vi "CRYCalcu Arithmetic Curve.vi"(4 "dB ref":dbl format="%#_6p", 6 "B data for units":T1={"Name"="", "Curve"=[], "X data"=1, "Y data"=1, "Z data"=1, "X axis"=0, "Y axis"=1, "Z axis"=1, "X unit"="Hz", "Y unit"="", "Z unit"="deg.", "X dB ref"=1.0, "Y dB ref"=1.0, "Z dB ref"=1.0, "single val"=FALSE, "protected"=FALSE, "display X"=TRUE, "display Y"=TRUE, "display Z"=TRUE, "Test Info"="", "Step No."=0, "Plot Settings"={"Color"=0, "Interpolation"=0, "Point Style"=0, "Line Style"=0, "Point Color"=0, "Line Width"=0, "Bar Plot Style"=0, "Fill To"=0}, "AutoProtect"=FALSE} {"Z data" items=["dB", "Lin"]; "X data" items=["dB", "Lin"]; "Y data" items=["dB", "Lin"]; "Z dB ref" format="%.1f"; "Z axis" items=["Log", "Lin"]; "X dB ref" format="%.1f"; "X axis" items=["Log", "Lin"]; "Y axis" items=["Log", "Lin"]; "Y dB ref" format="%.1f"; "Curve"."z" format="%.2f"; "Curve"."y" format="%.2f"; "Curve"."x" format="%.2f"}, 7 "A data for units":T1={"Name"="", "Curve"=[], "X data"=1, "Y data"=1, "Z data"=1, "X axis"=0, "Y axis"=1, "Z axis"=1, "X unit"="Hz", "Y unit"="", "Z unit"="deg.", "X dB ref"=1.0, "Y dB ref"=1.0, "Z dB ref"=1.0, "single val"=FALSE, "protected"=FALSE, "display X"=TRUE, "display Y"=TRUE, "display Z"=TRUE, "Test Info"="", "Step No."=0, "Plot Settings"={"Color"=0, "Interpolation"=0, "Point Style"=0, "Line Style"=0, "Point Color"=0, "Line Width"=0, "Bar Plot Style"=0, "Fill To"=0}, "AutoProtect"=FALSE} {"Z data" items=["dB", "Lin"]; "X data" items=["dB", "Lin"]; "Y data" items=["dB", "Lin"]; "Z dB ref" format="%.1f"; "Z axis" items=["Log", "Lin"]; "X dB ref" format="%.1f"; "X axis" items=["Log", "Lin"]; "Y axis" items=["Log", "Lin"]; "Y dB ref" format="%.1f"; "Curve"."z" format="%.2f"; "Curve"."y" format="%.2f"; "Curve"."x" format="%.2f"}, 8 "Curve B":cluster{"x":dbl, "y":dbl, "z":dbl}[](array[cluster]) {"z" format="%.2f"; "y" format="%.2f"; "x" format="%.2f"}, 9 "operator":u16(ring) items=["+", "--", "x", "/"], 10 "Work in":u16(slide), 11 "Curve A":cluster{"x":dbl, "y":dbl, "z":dbl}[](array[cluster]) {"z" format="%.2f"; "y" format="%.2f"; "x" format="%.2f"}) -> (2 "Result":cluster{"x":dbl, "y":dbl, "z":dbl}[](array[cluster]) {"z" format="%.2f"; "y" format="%.2f"; "x" format="%.2f"})   [LabVIEW 2013]
uses:
  Typedef Control/CRYData Cluster.ctl
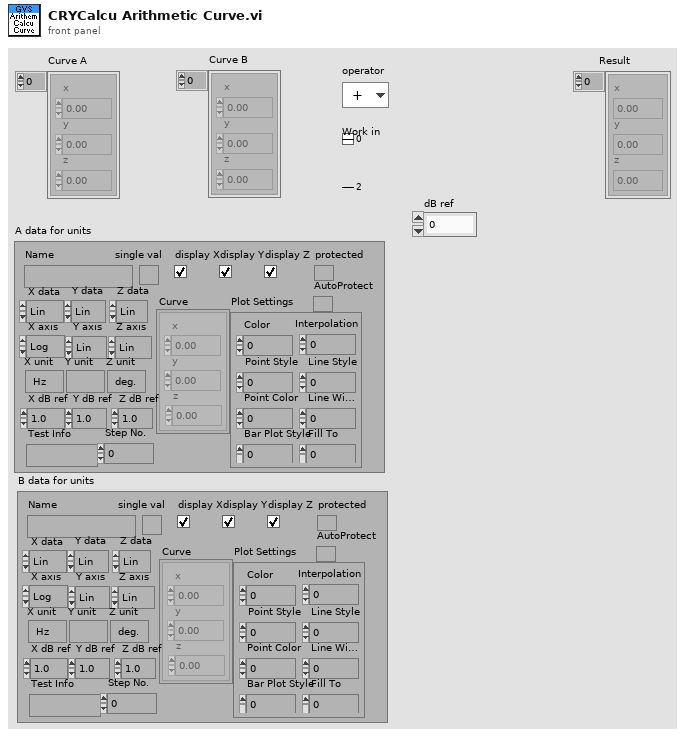
[diagram p1: front panel]
types:
  T1 = typedef "CRYData Cluster.ctl" = cluster{"Name":string, "Curve":cluster{"x":dbl, "y":dbl, "z":dbl}[], "X data":u16, "Y data":u16, "Z data":u16, "X axis":u16, "Y axis":u16, "Z axis":u16, "X unit":string, "Y unit":string, "Z unit":string, "X dB ref":dbl, "Y dB ref":dbl, "Z dB ref":dbl, "single val":bool, "protected":bool, "display X":bool, "display Y":bool, "display Z":bool, "Test Info":string, "Step No.":i32, "Plot Settings":cluster{"Color":u32, "Interpolation":u8, "Point Style":u8, "Line Style":u8, "Point Color":u32, "Line Width":u8, "Bar Plot Style":u8, "Fill To":i16}, "AutoProtect":bool}
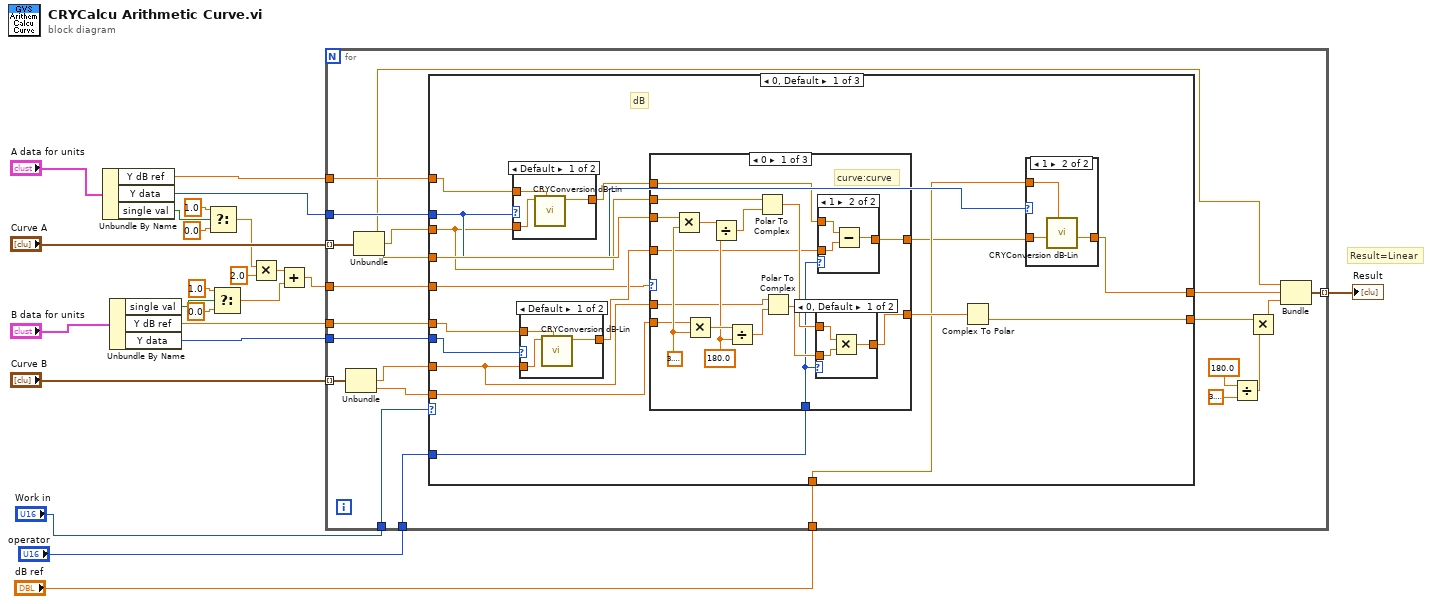
[diagram p0: block diagram]
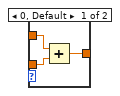
[diagram p2: hidden frame]
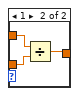
[diagram p3: hidden frame]
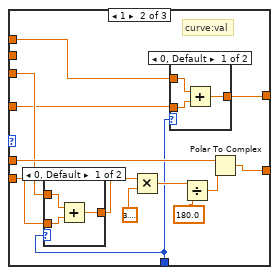
[diagram p4: hidden frame]
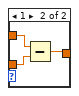
[diagram p5: hidden frame]
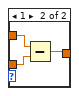
[diagram p6: hidden frame]
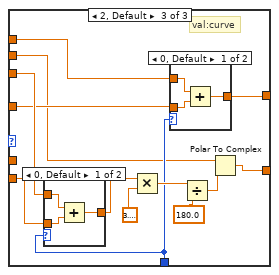
[diagram p7: hidden frame]
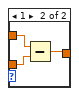
[diagram p8: hidden frame]
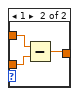
[diagram p9: hidden frame]
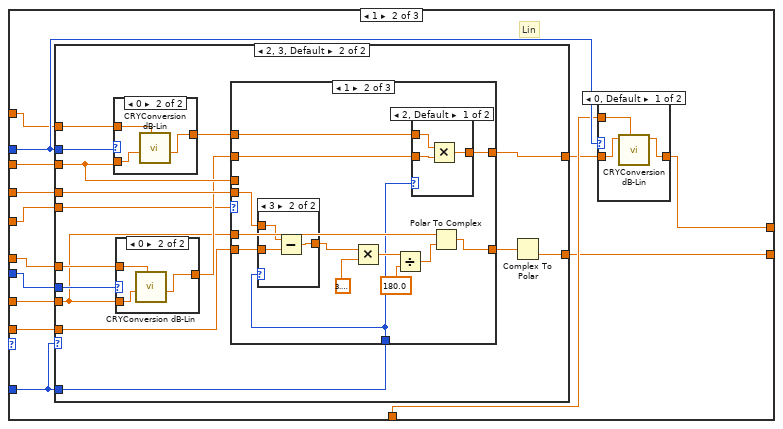
[diagram p13: hidden frame]
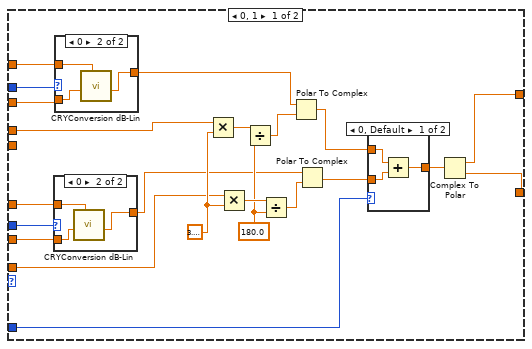
[diagram p14: hidden frame]
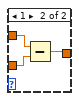
[diagram p15: hidden frame]
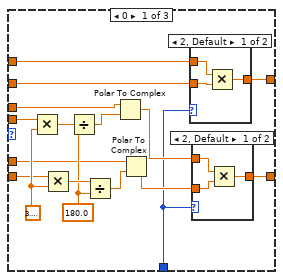
[diagram p18: hidden frame]
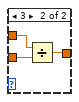
[diagram p19: hidden frame]
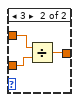
[diagram p20: hidden frame]
diagram:
  # "Result=Linear"
  n1 = Unbundle By Name("A data for units") -> ("Y dB ref"=w17:dbl, "Y data"=w18:u16, "single val"=w13:bool)
  n2 = Unbundle By Name("B data for units") -> ("single val"=w8:bool, "Y dB ref"=w15:dbl, "Y data"=w16:u16)
  n3 = Select(t=1.0, s=w13, f=0.0) -> (s? t:f=w7:dbl)
  n4 = Select(t=1.0, s=w8, f=0.0) -> (s? t:f=w5:dbl)
  n5 = Multiply(x=w7, y=2.0) -> (x*y=w6:dbl)
  n6 = Add(x=w6, y=w5) -> (x+y=w4:dbl)
  n7 = for {
    tunnel: "Curve B" -> [w45] mode=indexing
    tunnel: "Curve A" -> [w44] mode=indexing
    tunnel: [w43] -> w22 mode=indexing
    tunnel: "operator" -> [w42]
    tunnel: "Work in" -> [w41]
    tunnel: w18 -> [w40]
    tunnel: w17 -> [w39]
    tunnel: w16 -> [w38]
    tunnel: w15 -> [w37]
    tunnel: "dB ref" -> [w36]
    tunnel: w4 -> [w25]
    n8 = Unbundle(w45) -> ("y"=w34:dbl, "z"=w28:dbl)  [unwired: 1 out]
    n9 = Unbundle(w44) -> ("x"=w24:dbl, "y"=w35:dbl, "z"=w29:dbl)
    n10 = case shown="0, Default" w41 {
      tunnel: w35 -> [w49 w159 w315]
      tunnel: w34 -> [w51 w160 w314]
      tunnel: w42 -> [w52 w157 w316]
      tunnel: w40 -> [w57 w163 w312]
      tunnel: w39 -> [w56 w162 w318]
      tunnel: w38 -> [w61 w167 w323]
      tunnel: w37 -> [w60 w166 w322]
      tunnel: [w55 w161 w310] -> w33
      tunnel: w36 -> [w50 w158 w313]
      tunnel: w29 -> [w59 w165 w320]
      tunnel: w28 -> [w58 w164 w319]
      tunnel: [w54 w155 w317] -> w26
      tunnel: w25 -> [w47 w154 _]
      frame 0, Default {
        # "dB"
        n11 = case shown="Default" w57 {
          tunnel: w49 -> [w151 w153]
          tunnel: [w150 w153] -> w48
          tunnel: w56 -> [w152 _]
          frame Default {
            n12 = call "CRYConversion dB-Lin.vi"("dB ref."=w152, "Lin In"=w151) -> ("Log Out"=w150:dbl)  [unwired: 4 in, 3 out]
          }
          frame 0 {
          }
        }
        n13 = case shown="Default" w61 {
          tunnel: w51 -> [w147 w149]
          tunnel: [w146 w149] -> w53
          tunnel: w60 -> [w148 _]
          frame Default {
            n14 = call "CRYConversion dB-Lin.vi"("dB ref."=w148, "Lin In"=w147) -> ("Log Out"=w146:dbl)  [unwired: 4 in, 3 out]
          }
          frame 0 {
          }
        }
        n15 = case shown="0" w47 {
          tunnel: [w79 w96 w122] -> w62
          tunnel: w59 -> [w70 w99 w125]
          tunnel: w58 -> [w69 w98 w124]
          tunnel: w53 -> [w68 w94 w120]
          tunnel: [w67 w93 w119] -> w46
          tunnel: w52 -> [w66 w92 w118]
          tunnel: w51 -> [w65 w100 _]
          tunnel: w49 -> [w64 _ w117]
          tunnel: w48 -> [w63 w95 w121]
          frame 0 {
            w71 = 180.0
            w74 = 3.141592653589793
            # "curve:curve"
            n16 = Multiply(x=w70, y=w74) -> (x*y=w72:dbl)
            n17 = Multiply(x=w69, y=w74) -> (x*y=w73:dbl)
            n18 = Divide(x=w72, y=w71) -> (x/y=w75:dbl)
            n19 = Divide(x=w73, y=w71) -> (x/y=w76:dbl)
            n20 = Polar To Complex(1:w75, 2:w64) -> (0:w77:cdb)
            n21 = Polar To Complex(1:w76, 2:w65) -> (0:w78:cdb)
            n22 = case shown="0, Default" w66 {
              tunnel: [w86 w91] -> w79
              tunnel: w78 -> [w87 w89]
              tunnel: w77 -> [w88 w90]
              frame 0, Default {
                n23 = Multiply(x=w88, y=w87) -> (x*y=w86:cdb)
              }
              frame 1 {
                n24 = Divide(x=w90, y=w89) -> (x/y=w91:cdb)
              }
            }
            n25 = case shown="1" w66 {
              tunnel: [w80 w85] -> w67
              tunnel: w68 -> [w81 w83]
              tunnel: w63 -> [w82 w84]
              frame 0, Default {
                n26 = Add(x=w82, y=w81) -> (x+y=w80:dbl)
              }
              frame 1 {
                n27 = Subtract(x=w84, y=w83) -> (x-y=w85:dbl)
              }
            }
          }
          frame 1 {
            # "curve:val"
            n28 = case shown="0, Default" w92 {
              tunnel: [w111 w116] -> w97
              tunnel: w98 -> [w112 w114]
              tunnel: w99 -> [w113 w115]
              frame 0, Default {
                n29 = Add(x=w113, y=w112) -> (x+y=w111:dbl)
              }
              frame 1 {
                n30 = Subtract(x=w115, y=w114) -> (x-y=w116:dbl)
              }
            }
            n31 = Multiply(x=w97, y=3.141592653589793) -> (x*y=w102:dbl)
            n32 = case shown="0, Default" w92 {
              tunnel: [w105 w110] -> w93
              tunnel: w94 -> [w106 w108]
              tunnel: w95 -> [w107 w109]
              frame 0, Default {
                n33 = Add(x=w107, y=w106) -> (x+y=w105:dbl)
              }
              frame 1 {
                n34 = Subtract(x=w109, y=w108) -> (x-y=w110:dbl)
              }
            }
            n35 = Divide(x=w102, y=180.0) -> (x/y=w104:dbl)
            n36 = Polar To Complex(1:w104, 2:w100) -> (0:w96:cdb)
          }
          frame 2, Default {
            # "val:curve"
            n37 = case shown="0, Default" w118 {
              tunnel: [w136 w141] -> w123
              tunnel: w124 -> [w137 w139]
              tunnel: w125 -> [w138 w140]
              frame 0, Default {
                n38 = Add(x=w138, y=w137) -> (x+y=w136:dbl)
              }
              frame 1 {
                n39 = Subtract(x=w140, y=w139) -> (x-y=w141:dbl)
              }
            }
            n40 = Multiply(x=w123, y=3.141592653589793) -> (x*y=w127:dbl)
            n41 = case shown="0, Default" w118 {
              tunnel: [w130 w135] -> w119
              tunnel: w120 -> [w131 w133]
              tunnel: w121 -> [w132 w134]
              frame 0, Default {
                n42 = Add(x=w132, y=w131) -> (x+y=w130:dbl)
              }
              frame 1 {
                n43 = Subtract(x=w134, y=w133) -> (x-y=w135:dbl)
              }
            }
            n44 = Divide(x=w127, y=180.0) -> (x/y=w129:dbl)
            n45 = Polar To Complex(1:w129, 2:w117) -> (0:w122:cdb)
          }
        }
        n46 = Complex To Polar(r * e^(i*theta)=w62) -> (theta=w54:dbl)  [unwired: 1 out]
        n47 = case shown="1" w57 {
          tunnel: w46 -> [w142 w145]
          tunnel: [w142 w144] -> w55
          tunnel: w50 -> [_ w143]
          frame 0, Default {
          }
          frame 1 {
            n48 = call "CRYConversion dB-Lin.vi"("dB ref."=w143, "Log In"=w145) -> ("Lin Out"=w144:dbl)  [unwired: 4 in, 3 out]
          }
        }
      }
      frame 1 {
        # "Lin"
        n49 = case shown="2, 3, Default" w157 {
          tunnel: [w169 w205] -> w155
          tunnel: w167 -> [w181 w218]
          tunnel: w166 -> [w180 w217]
          tunnel: w165 -> [w179 w216]
          tunnel: w164 -> [w178 w215]
          tunnel: w163 -> [w177 w214]
          tunnel: w162 -> [w176 w213]
          tunnel: w160 -> [w175 w209]
          tunnel: w159 -> [w174 w211]
          tunnel: w157 -> [w173 w207]
          tunnel: [w168 w208] -> w156
          tunnel: w154 -> [_ w204]
          frame 0, 1 {
            w182 = 180.0
            w185 = 3.141592653589793
            n50 = case shown="0" w181 {
              tunnel: w175 -> [w196 w198]
              tunnel: [w196 w197] -> w172
              tunnel: w180 -> [_ w199]
              frame Default {
              }
              frame 0 {
                n51 = call "CRYConversion dB-Lin.vi"("dB ref."=w199, "Log In"=w198) -> ("Lin Out"=w197:dbl)  [unwired: 4 in, 3 out]
              }
            }
            n52 = case shown="0" w177 {
              tunnel: w174 -> [w200 w202]
              tunnel: [w200 w201] -> w171
              tunnel: w176 -> [_ w203]
              frame Default {
              }
              frame 0 {
                n53 = call "CRYConversion dB-Lin.vi"("dB ref."=w203, "Log In"=w202) -> ("Lin Out"=w201:dbl)  [unwired: 4 in, 3 out]
              }
            }
            n54 = Multiply(x=w179, y=w185) -> (x*y=w183:dbl)
            n55 = Multiply(x=w178, y=w185) -> (x*y=w184:dbl)
            n56 = Divide(x=w183, y=w182) -> (x/y=w186:dbl)
            n57 = Divide(x=w184, y=w182) -> (x/y=w187:dbl)
            n58 = Polar To Complex(1:w186, 2:w171) -> (0:w188:cdb)
            n59 = Polar To Complex(1:w187, 2:w172) -> (0:w189:cdb)
            n60 = case shown="0, Default" w173 {
              tunnel: [w190 w195] -> w170
              tunnel: w189 -> [w191 w193]
              tunnel: w188 -> [w192 w194]
              frame 0, Default {
                n61 = Add(x=w192, y=w191) -> (x+y=w190:cdb)
              }
              frame 1 {
                n62 = Subtract(x=w194, y=w193) -> (x-y=w195:cdb)
              }
            }
            n63 = Complex To Polar(r * e^(i*theta)=w170) -> (r=w168:dbl, theta=w169:dbl)
          }
          frame 2, 3, Default {
            n64 = case shown="0" w214 {
              tunnel: w211 -> [w302 w304]
              tunnel: [w302 w303] -> w212
              tunnel: w213 -> [_ w305]
              frame Default {
              }
              frame 0 {
                n65 = call "CRYConversion dB-Lin.vi"("dB ref."=w305, "Log In"=w304) -> ("Lin Out"=w303:dbl)  [unwired: 4 in, 3 out]
              }
            }
            n66 = case shown="0" w218 {
              tunnel: w209 -> [w298 w300]
              tunnel: [w298 w299] -> w210
              tunnel: w217 -> [_ w301]
              frame Default {
              }
              frame 0 {
                n67 = call "CRYConversion dB-Lin.vi"("dB ref."=w301, "Log In"=w300) -> ("Lin Out"=w299:dbl)  [unwired: 4 in, 3 out]
              }
            }
            n68 = case shown="1" w204 {
              tunnel: w216 -> [w227 w249 w275]
              tunnel: w215 -> [w226 w251 w277]
              tunnel: w212 -> [w225 w256 w281]
              tunnel: w211 -> [w224 _ w274]
              tunnel: w210 -> [w223 w255 w280]
              tunnel: w209 -> [w222 w254 _]
              tunnel: [w221 w253 w279] -> w208
              tunnel: w207 -> [w220 w248 w273]
              tunnel: [w219 w252 w278] -> w206
              frame 0 {
                w228 = 180.0
                w231 = 3.141592653589793
                n69 = Multiply(x=w227, y=w231) -> (x*y=w229:dbl)
                n70 = Multiply(x=w226, y=w231) -> (x*y=w230:dbl)
                n71 = Divide(x=w229, y=w228) -> (x/y=w232:dbl)
                n72 = Divide(x=w230, y=w228) -> (x/y=w233:dbl)
                n73 = Polar To Complex(1:w232, 2:w224) -> (0:w234:cdb)
                n74 = Polar To Complex(1:w233, 2:w222) -> (0:w235:cdb)
                n75 = case shown="2, Default" w220 {
                  tunnel: [w236 w241] -> w221
                  tunnel: w223 -> [w237 w239]
                  tunnel: w225 -> [w238 w240]
                  frame 2, Default {
                    n76 = Multiply(x=w238, y=w237) -> (x*y=w236:dbl)
                  }
                  frame 3 {
                    n77 = Divide(x=w240, y=w239) -> (x/y=w241:dbl)
                  }
                }
                n78 = case shown="2, Default" w220 {
                  tunnel: [w242 w247] -> w219
                  tunnel: w235 -> [w243 w245]
                  tunnel: w234 -> [w244 w246]
                  frame 2, Default {
                    n79 = Multiply(x=w244, y=w243) -> (x*y=w242:cdb)
                  }
                  frame 3 {
                    n80 = Divide(x=w246, y=w245) -> (x/y=w247:cdb)
                  }
                }
              }
              frame 1 {
                n81 = case shown="3" w248 {
                  tunnel: [w261 w266] -> w250
                  tunnel: w251 -> [w262 w264]
                  tunnel: w249 -> [w263 w265]
                  frame 2, Default {
                    n82 = Add(x=w263, y=w262) -> (x+y=w261:dbl)
                  }
                  frame 3 {
                    n83 = Subtract(x=w265, y=w264) -> (x-y=w266:dbl)
                  }
                }
                n84 = Multiply(x=w250, y=3.141592653589793) -> (x*y=w258:dbl)
                n85 = Divide(x=w258, y=180.0) -> (x/y=w260:dbl)
                n86 = case shown="2, Default" w248 {
                  tunnel: [w267 w272] -> w253
                  tunnel: w255 -> [w268 w270]
                  tunnel: w256 -> [w269 w271]
                  frame 2, Default {
                    n87 = Multiply(x=w269, y=w268) -> (x*y=w267:dbl)
                  }
                  frame 3 {
                    n88 = Divide(x=w271, y=w270) -> (x/y=w272:dbl)
                  }
                }
                n89 = Polar To Complex(1:w260, 2:w254) -> (0:w252:cdb)
              }
              frame 2, Default {
                n90 = case shown="3" w273 {
                  tunnel: [w286 w291] -> w276
                  tunnel: w277 -> [w287 w289]
                  tunnel: w275 -> [w288 w290]
                  frame 2, Default {
                    n91 = Add(x=w288, y=w287) -> (x+y=w286:dbl)
                  }
                  frame 3 {
                    n92 = Subtract(x=w290, y=w289) -> (x-y=w291:dbl)
                  }
                }
                n93 = Multiply(x=w276, y=3.141592653589793) -> (x*y=w283:dbl)
                n94 = Divide(x=w283, y=180.0) -> (x/y=w285:dbl)
                n95 = case shown="2, Default" w273 {
                  tunnel: [w292 w297] -> w279
                  tunnel: w280 -> [w293 w295]
                  tunnel: w281 -> [w294 w296]
                  frame 2, Default {
                    n96 = Multiply(x=w294, y=w293) -> (x*y=w292:dbl)
                  }
                  frame 3 {
                    n97 = Divide(x=w296, y=w295) -> (x/y=w297:dbl)
                  }
                }
                n98 = Polar To Complex(1:w285, 2:w274) -> (0:w278:cdb)
              }
            }
            n99 = Complex To Polar(r * e^(i*theta)=w206) -> (theta=w205:dbl)  [unwired: 1 out]
          }
        }
        n100 = case shown="0, Default" w163 {
          tunnel: w156 -> [w307 w309]
          tunnel: [w306 w309] -> w161
          tunnel: w158 -> [w308 _]
          frame 0, Default {
            n101 = call "CRYConversion dB-Lin.vi"("dB ref."=w308, "Lin In"=w307) -> ("Log Out"=w306:dbl)  [unwired: 4 in, 3 out]
          }
          frame 1 {
          }
        }
      }
      frame 2 {
        # "pow"
        n102 = case shown="0" w323 {
          tunnel: w314 -> [w396 w398]
          tunnel: [w396 w397] -> w321
          tunnel: w322 -> [_ w399]
          frame Default {
          }
          frame 0 {
            n103 = call "CRYConversion dB-Lin.vi"("dB ref."=w399, "Log In"=w398) -> ("Lin Out"=w397:dbl)  [unwired: 4 in, 3 out]
          }
        }
        n104 = case shown="0" w312 {
          tunnel: w315 -> [w400 w402]
          tunnel: [w400 w401] -> w324
          tunnel: w318 -> [_ w403]
          frame Default {
          }
          frame 0 {
            n105 = call "CRYConversion dB-Lin.vi"("dB ref."=w403, "Log In"=w402) -> ("Lin Out"=w401:dbl)  [unwired: 4 in, 3 out]
          }
        }
        n106 = case shown="0, 1, Default" w316 {
          tunnel: w324 -> [w335 w367]
          tunnel: w321 -> [w334 w366]
          tunnel: w320 -> [w333 w370]
          tunnel: w319 -> [w332 w369]
          tunnel: w316 -> [w331 w362]
          tunnel: [w330 w368] -> w317
          tunnel: w315 -> [_ w365]
          tunnel: w314 -> [_ w364]
          tunnel: [w329 w363] -> w311
          frame 0, 1, Default {
            w336 = 180.0
            w339 = 3.141592653589793
            n107 = Multiply(x=w333, y=w339) -> (x*y=w337:dbl)
            n108 = Multiply(x=w332, y=w339) -> (x*y=w338:dbl)
            n109 = Divide(x=w337, y=w336) -> (x/y=w340:dbl)
            n110 = Divide(x=w338, y=w336) -> (x/y=w341:dbl)
            n111 = Polar To Complex(1:w340, 2:w335) -> (0:w342:cdb)
            n112 = Polar To Complex(1:w341, 2:w334) -> (0:w343:cdb)
            n113 = case shown="0, Default" w331 {
              tunnel: [w345 w354] -> w344
              tunnel: w343 -> [w346 w356]
              tunnel: w342 -> [w347 w355]
              frame 0, Default {
                # "+"
                n114 = Complex To Polar(r * e^(i*theta)=w346) -> (r=w348:dbl)  [unwired: 1 out]
                n115 = Complex To Polar(r * e^(i*theta)=w347) -> (r=w349:dbl)  [unwired: 1 out]
                n116 = Square(x=w349) -> (x^2=w352:dbl)
                n117 = Square(x=w348) -> (x^2=w351:dbl)
                n118 = Add(x=w352, y=w351) -> (x+y=w350:dbl)
                n119 = Square Root(x=w350) -> (sqrt(x)=w345:dbl)
              }
              frame 1 {
                n120 = Complex To Polar(r * e^(i*theta)=w356) -> (r=w358:dbl)  [unwired: 1 out]
                n121 = Complex To Polar(r * e^(i*theta)=w355) -> (r=w353:dbl)  [unwired: 1 out]
                n122 = Square(x=w353) -> (x^2=w361:dbl)
                n123 = Square(x=w358) -> (x^2=w360:dbl)
                n124 = Subtract(x=w361, y=w360) -> (x-y=w359:dbl)
                n125 = Absolute Value(x=w359) -> (abs(x)=w357:dbl)
                n126 = Square Root(x=w357) -> (sqrt(x)=w354:dbl)
              }
            }
            n127 = Complex To Polar(r * e^(i*theta)=w344) -> (r=w329:dbl, theta=w330:dbl)
          }
          frame 2, 3 {
            w371 = 180.0
            w374 = 3.141592653589793
            n128 = Multiply(x=w370, y=w374) -> (x*y=w372:dbl)
            n129 = Multiply(x=w369, y=w374) -> (x*y=w373:dbl)
            n130 = Divide(x=w372, y=w371) -> (x/y=w375:dbl)
            n131 = Divide(x=w373, y=w371) -> (x/y=w376:dbl)
            n132 = Polar To Complex(1:w375, 2:w365) -> (0:w377:cdb)
            n133 = Polar To Complex(1:w376, 2:w364) -> (0:w378:cdb)
            n134 = case shown="3" w362 {
              tunnel: [w386 w391] -> w379
              tunnel: w378 -> [w387 w393]
              tunnel: w377 -> [w388 w392]
              frame 2, Default {
                n135 = Complex To Polar(r * e^(i*theta)=w388) -> (r=w390:dbl)  [unwired: 1 out]
                n136 = Complex To Polar(r * e^(i*theta)=w387) -> (r=w389:dbl)  [unwired: 1 out]
                n137 = Multiply(x=w390, y=w389) -> (x*y=w386:dbl)
              }
              frame 3 {
                n138 = Complex To Polar(r * e^(i*theta)=w392) -> (r=w394:dbl)  [unwired: 1 out]
                n139 = Complex To Polar(r * e^(i*theta)=w393) -> (r=w395:dbl)  [unwired: 1 out]
                n140 = Divide(x=w394, y=w395) -> (x/y=w391:dbl)
              }
            }
            n141 = case shown="2, Default" w362 {
              tunnel: [w382 w385] -> w363
              tunnel: w367 -> [w381 w384]
              tunnel: w366 -> [w380 w383]
              frame 2, Default {
                n142 = Multiply(x=w381, y=w380) -> (x*y=w382:dbl)
              }
              frame 3 {
                n143 = Divide(x=w384, y=w383) -> (x/y=w385:dbl)
              }
            }
            n144 = Complex To Polar(r * e^(i*theta)=w379) -> (theta=w368:dbl)  [unwired: 1 out]
          }
        }
        n145 = case shown="0, Default" w312 {
          tunnel: w311 -> [w326 w328]
          tunnel: [w325 w328] -> w310
          tunnel: w313 -> [w327 _]
          frame 0, Default {
            n146 = call "CRYConversion dB-Lin.vi"("dB ref."=w327, "Lin In"=w326) -> ("Log Out"=w325:dbl)  [unwired: 4 in, 3 out]
          }
          frame 1 {
          }
        }
      }
    }
    n147 = Divide(x=180.0, y=3.141592653589793) -> (x/y=w27:dbl)
    n148 = Multiply(x=w26, y=w27) -> (x*y=w30:dbl)
    n149 = Bundle("x"=w24, "Log Out"=w33, w30) -> (w43:cluster{"x":dbl, "Log Out":dbl, dbl})  [unwired: 1 in]
  }
  "Result" <- w22
